vi "item select new ref.vi"(8 "error in (no error)":errorcluster, 11 "Listbox or Tree":refnum<vi>) -> (0 "error out":errorcluster, 3 "Loop data":T1)   [LabVIEW 2020, in "UI_ItemSelect_OpenSource.lvlib"]
uses:
  UI_ItemSelect_OpenSource.lvlib
  Tree item select loop data.ctl
  Item select ref type.ctl
  Tree item loop data.ctl
  Tree item selection indices.ctl
  checkbox state.ctl
  item select tree lock states.ctl
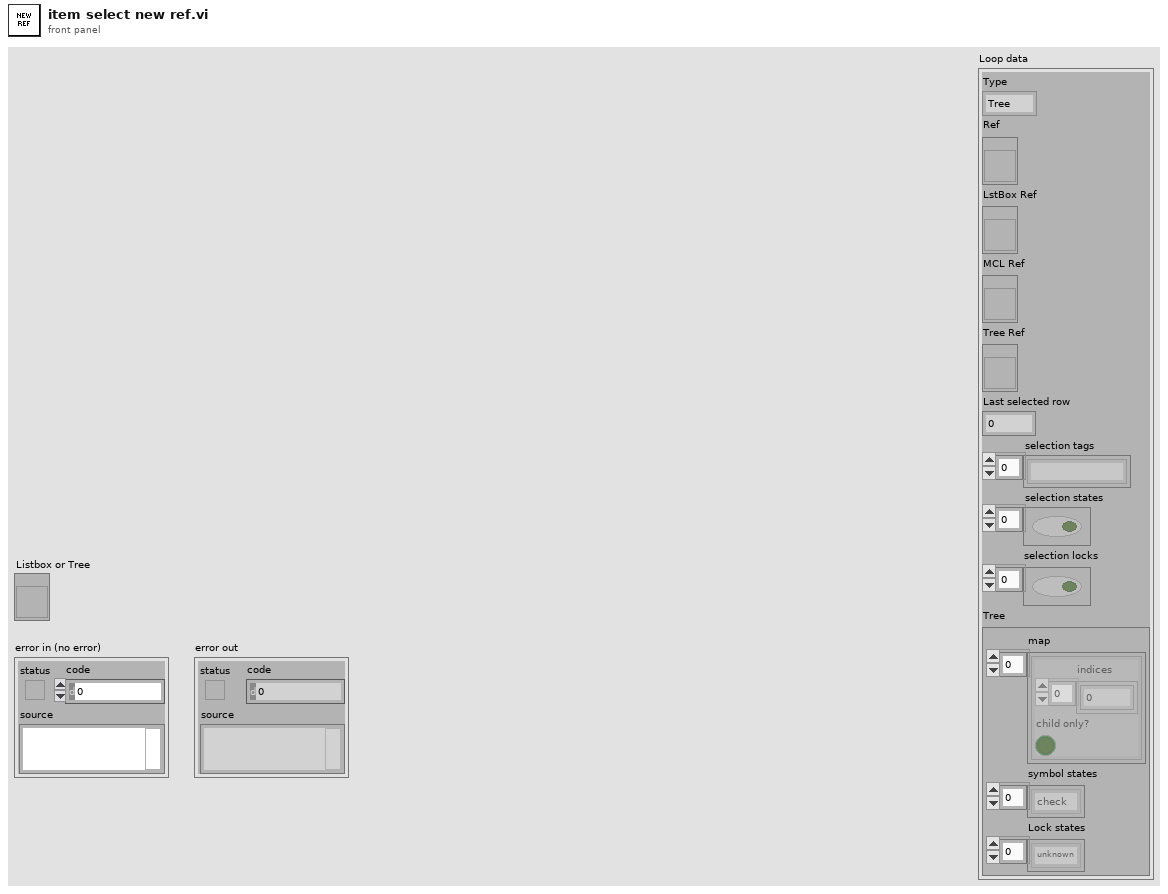
[diagram p1: front panel]
types:
  T1 = typedef "UI_ItemSelect_OpenSource.lvlib/Tree item select loop data.ctl" = cluster{"Type":T2, "Ref":refnum<vi>, "LstBox Ref":refnum<vi>, "MCL Ref":refnum<vi>, "Tree Ref":refnum<vi>, "Last selected row":i32, "selection tags":string[], "selection states":bool[], "selection locks":bool[], "Tree":T3}
  T2 = typedef "UI_ItemSelect_OpenSource.lvlib/Item select ref type.ctl" = enum16{"Tree", "MCL", "ListBox"}
  T3 = typedef "UI_ItemSelect_OpenSource.lvlib/Tree item loop data.ctl" = cluster{"map":T4[], "symbol states":T5[], "Lock states":T6[]}
  T4 = typedef "UI_ItemSelect_OpenSource.lvlib/Tree item selection indices.ctl" = cluster{"indices":i32[], "child only?":bool}
  T5 = typedef "UI_ItemSelect_OpenSource.lvlib/checkbox state.ctl" = enum16{"unknown", "check", "some", "no check"}
  T6 = typedef "UI_ItemSelect_OpenSource.lvlib/item select tree lock states.ctl" = enum16{"unknown", "locked", "unlocked"}
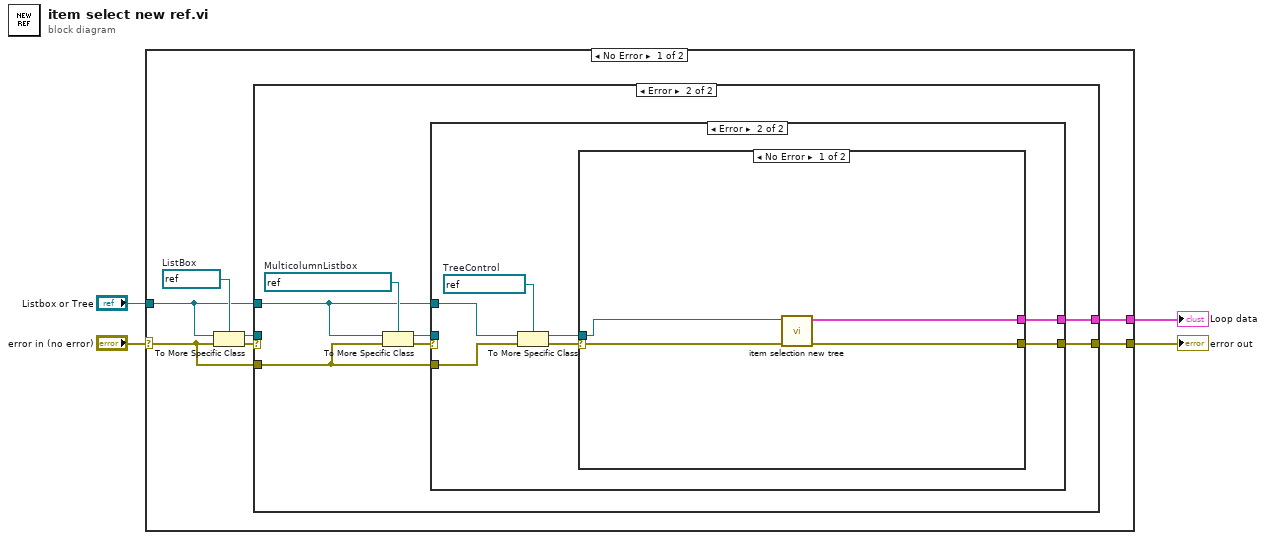
[diagram p0: block diagram]
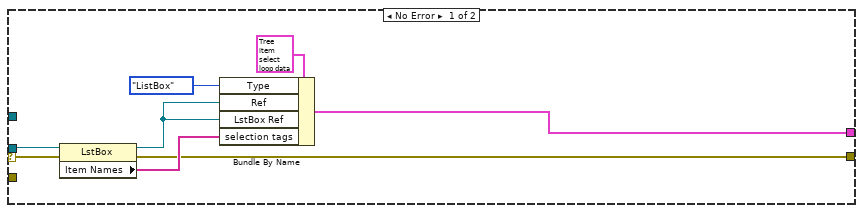
[diagram p2: hidden frame]
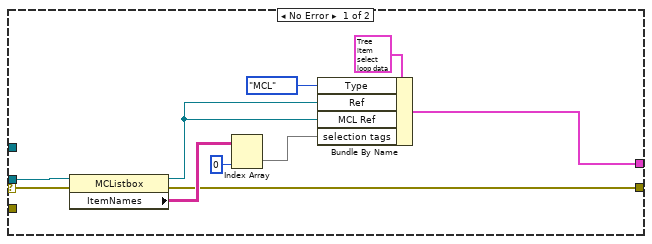
[diagram p3: hidden frame]
diagram:
  n1 = case shown="No Error" "error in (no error)" {
    selector: "error in (no error)" -> [w8 w49]
    tunnel: [w6 w49] -> w3
    tunnel: "Listbox or Tree" -> [w7 _]
    tunnel: [w5 _] -> w1
    frame No Error {
      w11 = refnum<vi> refnum  # ListBox
      n2 = To More Specific Class(target class=w11, reference=w7, error in=w8) -> (specific class reference=w9:refnum<vi>, error out=w10:errorcluster)
      n3 = case shown="Error" w10 {
        selector: w10 -> [w17 _]
        tunnel: w9 -> [w16 _]
        tunnel: w8 -> [_ w22]
        tunnel: w7 -> [_ w23]
        tunnel: [w13 w21] -> w6
        tunnel: [w14 w20] -> w5
        frame No Error {
          n4 = property class="LstBox"(reference=w16, error in=w17) -> (reference out=w12:refnum<vi>, error out=w13:errorcluster, "Item Names"=w15:string[])
          n5 = Bundle By Name(cluster=T1 {"Type"=enum."Tree", "Ref"=refnum, "LstBox Ref"=refnum, "MCL Ref"=refnum, "Tree Ref"=refnum, "Last selected row"=0, "selection tags"=[], "selection states"=[], "selection locks"=[], "Tree"={"map"=[], "symbol states"=[], "Lock states"=[]}} ("Loop data"), "Type"=Item_select_ref_type."ListBox", "Ref"=w12, "LstBox Ref"=w12, "selection tags"=w15) -> (w14:T1)
        }
        frame Error {
          w26 = refnum<vi> refnum  # MulticolumnListbox
          n6 = To More Specific Class(target class=w26, reference=w23, error in=w22) -> (specific class reference=w24:refnum<vi>, error out=w25:errorcluster)
          n7 = case shown="Error" w25 {
            selector: w25 -> [w29 _]
            tunnel: w24 -> [w33 _]
            tunnel: w23 -> [_ w42]
            tunnel: w22 -> [_ w41]
            tunnel: [w28 w38] -> w21
            tunnel: [w34 w37] -> w20
            frame No Error {
              n8 = property class="MCListbox"(reference=w33, error in=w29) -> (reference out=w27:refnum<vi>, error out=w28:errorcluster, "ItemNames"=w32:string[][])
              n9 = Index Array(array=w32, index (col)=0 ("disabled index (col)")) -> (element=w30:string[])  [unwired: 1 in]
              n10 = Bundle By Name(cluster=T1 {"Type"=enum."Tree", "Ref"=refnum, "LstBox Ref"=refnum, "MCL Ref"=refnum, "Tree Ref"=refnum, "Last selected row"=0, "selection tags"=[], "selection states"=[], "selection locks"=[], "Tree"={"map"=[], "symbol states"=[], "Lock states"=[]}} ("Loop data"), "Type"=Item_select_ref_type."MCL", "Ref"=w27, "MCL Ref"=w27, "selection tags"=w30) -> (w34:T1)
            }
            frame Error {
              w43 = refnum<vi> refnum  # TreeControl
              n11 = To More Specific Class(target class=w43, reference=w42, error in=w41) -> (specific class reference=w40:refnum<vi>, error out=w39:errorcluster)
              n12 = case shown="No Error" w39 {
                selector: w39 -> [w46 w48]
                tunnel: w40 -> [w47 _]
                tunnel: [w45 w48] -> w38
                tunnel: [w44 _] -> w37
                frame No Error {
                  n13 = call "item selection new tree.vi"("error in (no error)"=w46, "Tree ref"=w47) -> ("error out"=w45:errorcluster, "Loop data"=w44:T1)  [unwired: 8 in]
                }
                frame Error {
                }
              }
            }
          }
        }
      }
    }
    frame Error {
    }
  }
  "Loop data" <- w1
  "error out" <- w3
